vi "Create New Bucket.vi"() -> ()   [LabVIEW 2015]
doc: "Demonstrates the use of the <b>Create Bucket</b> VI in the LabVIEW Interface for Amazon S3 toolkit."
uses:
  Core/HTTP Request/Region.ctl
  Core/HTTP Request/AWS Credentials.ctl
  Bucket/Bucket.lvclass
  Core/HTTP Request/HTTP Request.lvclass
panel:
  in  "Secret Key":string
  in  "Access Key":string
  in  "Bucket Name":string
  in  "Region":T1
  # "Overview: Demonstrates how to create a new Amazon S3 bucket.\nRequirements: LabVIEW AWS Toolkit and a registered Amazon AWS account\nInstructions:\n1. Specify the Access Key and Secret Key for your AWS account. You can create an account at http://aws.amazon.com.\n2. Specify Bucket Name for the bucket you want to create. Note that the bucket name must be globally unique.\n3. Run the VI. Verify in the Amazon S3 console that the specified bucket was created."
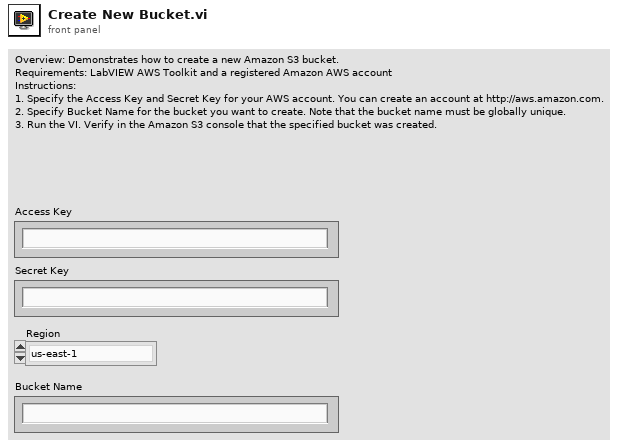
[diagram p1: front panel]
types:
  T1 = typedef "NI_AWS_Core.lvlib/HTTP Request.lvclass/Region.ctl" = enum16{"us-east-1", "us-east-2", "us-west-1", "us-west-2", "ap-northeast-1", "ap-northeast-2", "ap-southeast-1", "ap-southeast-2", "ca-central-1", "eu-central-1", "eu-west-1", "eu-west-2", "sa-east-1"}
  T2 = typedef "NI_AWS_Core.lvlib/HTTP Request.lvclass/AWS Credentials.ctl" = cluster{"Access Key":string, "Secret Key":string}
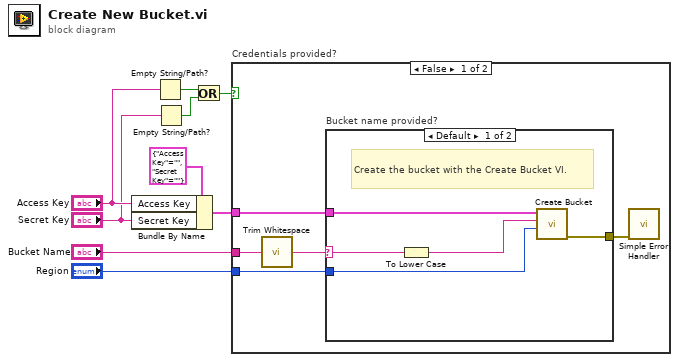
[diagram p0: block diagram]
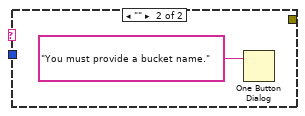
[diagram p2: hidden frame]
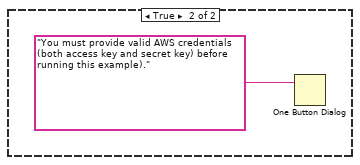
[diagram p3: hidden frame]
diagram:
  n1 = Bundle By Name(cluster=T2 {"Access Key"="", "Secret Key"=""} ("AWS Credentials in"), "Access Key"="Access Key", "Secret Key"="Secret Key") -> (w8:T2)
  n2 = Empty String/Path?(string/path="Access Key") -> (empty?=w7:bool)
  n3 = Empty String/Path?(string/path="Secret Key") -> (empty?=w5:bool)
  n4 = Or(x=w7, y=w5) -> (x .or. y?=w6:bool)
  n5 = case "Credentials provided?" shown="False" w6 {
    tunnel: w8 -> [w14 _]
    tunnel: "Bucket Name" -> [w12 _]
    tunnel: "Region" -> [w10 _]
    frame False {
      n6 = call <vilib>:"Trim Whitespace.vi"("string"=w12) -> ("trimmed string"=w11:string)  [unwired: 1 in]
      n7 = case "Bucket name provided?" shown="Default" w11 {
        selector: w11 -> [w19 _]
        tunnel: w14 -> [w15 _]
        tunnel: [w18 _] -> w13
        tunnel: w10 -> [w16 _]
        frame Default {
          # "Create the bucket with the Create Bucket VI."
          n8 = To Lower Case(string=w19) -> (all lower case string=w17:string)
          n9 = call "Create Bucket.vi"("Region"=w16, "Name"=w17, "AWS Credentials"=w15) -> ("error out"=w18:errorcluster)  [unwired: 7 in, 1 out]
        }
        frame "" {
          n10 = One Button Dialog(message="You must provide a bucket name.") -> ()  [unwired: 1 in, 1 out]
        }
      }
      n11 = call <vilib>:"Simple Error Handler.vi"("error in (no error)"=w13) -> ()  [unwired: 4 in, 5 out]
    }
    frame True {
      n12 = One Button Dialog(message="You must provide valid AWS credentials (both access key and secret key) before running this example).") -> ()  [unwired: 1 in, 1 out]
    }
  }
